vi "Query Retardation in Wave Units.vi"(8 "error in (no error)":errorcluster, 11 "VISA resource name":refnum<visa-resource-name>="COM1") -> (0 "error out":errorcluster, 2 "Fraction of wave Retardation":dbl, 3 "VISA resource name out":refnum<visa-resource-name>)   [LabVIEW 2017]
panel:
  out "read buffer":string
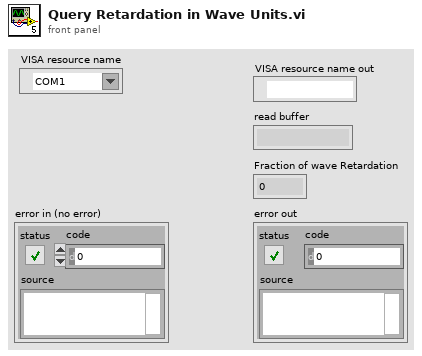
[diagram p1: front panel]
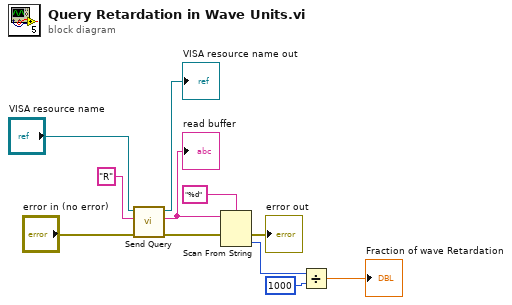
[diagram p0: block diagram]
diagram:
  n1 = call "Send Query.vi"("error in (no error)"="error in (no error)", "query string"="R" ("write buffer"), "VISA resource name"="VISA resource name") -> ("error out"=w3:errorcluster, "query output"=w1:string, "VISA resource name out"=→"VISA resource name out":refnum<visa-resource-name>)  [unwired: 6 in]
  "read buffer" <- w1
  n2 = Scan From String(format string="%d", input string=w1, error in=w3) -> (error out=→"error out":errorcluster, output 1=w10:i32)  [unwired: 2 in, 2 out]
  n3 = Divide(x=w10, y=1000) -> (x/y=→"Fraction of wave Retardation":dbl)
